vi "Extra Specialization Scripting VI Type.vi"(8 "error in (no error)":errorcluster, 10 "Element Type":variant, 11 "LVLibrary in":refnum<vi>) -> (0 "error out":errorcluster)   [LabVIEW 2020, in "FlexBlocks.lvlib"]
uses:
  FlexBlocks.lvlib
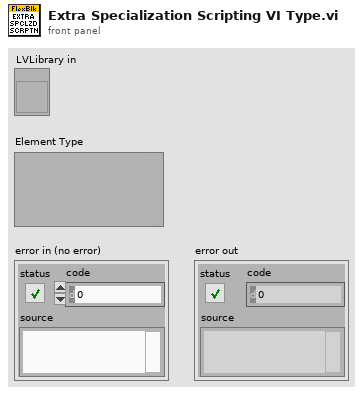
[diagram p1: front panel]
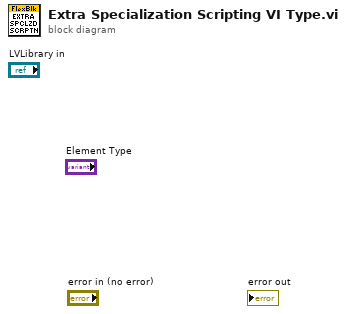
[diagram p0: block diagram]
diagram:
